vi "svx_Polar_Get_Attribute_String.vi"(4 "SVMS attribute":T1 items=["Pulse / Revolution", "Slope", "Threshold", "Hysteresis", "Order", "Reference Label", "Rotation Direction", "Pair String", "Polar Plot Type", "Sample Per Revolution", "Probe Angle", "Probe Angle X", "Probe Angle Y", "X Axis Unit", "OTB Plot Type"]) -> (1 "attribute name":string)   [LabVIEW 2017, in "SVX Polar Plot.xctl"]
uses:
  <vilib>/addons/_XControls/Polar Plot/SVX Polar Plot.xctl
  <vilib>/addons/_XControls/Polar Plot/subVIs/svx_Polar_Attribute.ctl
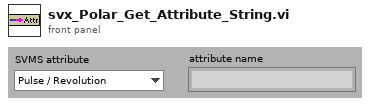
[diagram p1: front panel]
types:
  T1 = typedef "SVX Polar Plot.xctl/svx_Polar_Attribute.ctl" = u16
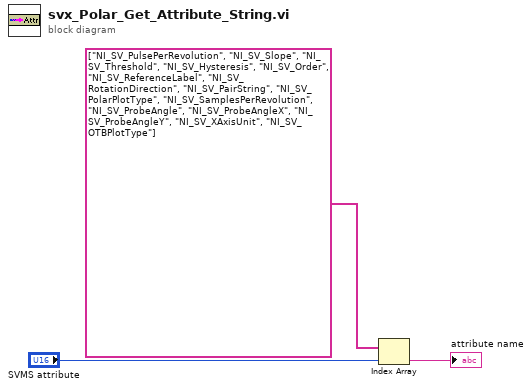
[diagram p0: block diagram]
diagram:
  n1 = Index Array(array=string[] ["NI_SV_PulsePerRevolution", "NI_SV_Slope", "NI_SV_Threshold", "NI_SV_Hysteresis", "NI_SV_Order", "NI_SV_ReferenceLabel", "NI_SV_RotationDirection", "NI_SV_PairString", "NI_SV_PolarPlotType", "NI_SV_SamplesPerRevolution", "NI_SV_ProbeAngle", "NI_SV_ProbeAngleX", "NI_SV_ProbeAngleY", "NI_SV_XAxisUnit", "NI_SV_OTBPlotType"], index="SVMS attribute") -> (element=→"attribute name":string)
